vi "Read configuration.vi"(8 "error in":errorcluster, 11 "Bus in":refnum<class "Bus.lvclass">) -> (0 "error out":errorcluster, 2 "configuration":refnum<class "NISE_CEF_serializable configuration.lvclass">, 3 "Bus out":refnum<class "Bus.lvclass">)   [LabVIEW 2014, in "Bus.lvclass"]
uses:
  Bus.lvclass
  <vilib>/NI/Configuration Framework/serializable configuration/NISE_CEF_serializable configuration.lvclass
  Bus.lvclass/Bus.ctl
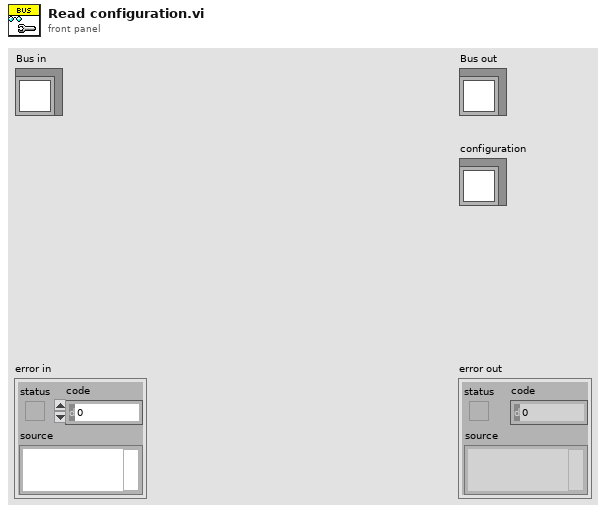
[diagram p1: front panel]
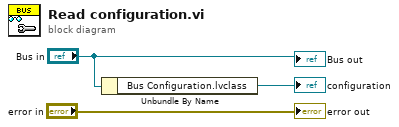
[diagram p0: block diagram]
diagram:
  n1 = Unbundle By Name("Bus in") -> ("Bus Configuration.lvclass"=→"configuration":refnum<class "Bus Configuration.lvclass">)
  "error out" <- "error in"
  "Bus out" <- "Bus in"
